vi "escalon_lab2.vi"() -> ()   [LabVIEW 2025]
uses:
  <vilib>/Utility/file.llb/Write Delimited Spreadsheet (DBL).vi
panel:
  out "Numeric 2":dbl
  out "Numeric":dbl
  in  "DC":dbl
  out "Waveform Chart":dynamicdata(graph)
  out "Thermometer":dbl(slide) scale=0.0..100.0
  in  "stop":bool
  # "Duty Cycle [%]"
  # "ALTO:"
  # "BAJO:"
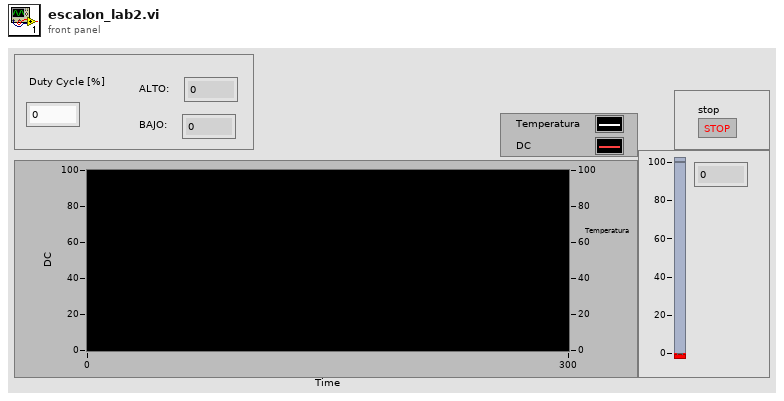
[diagram p1: front panel]
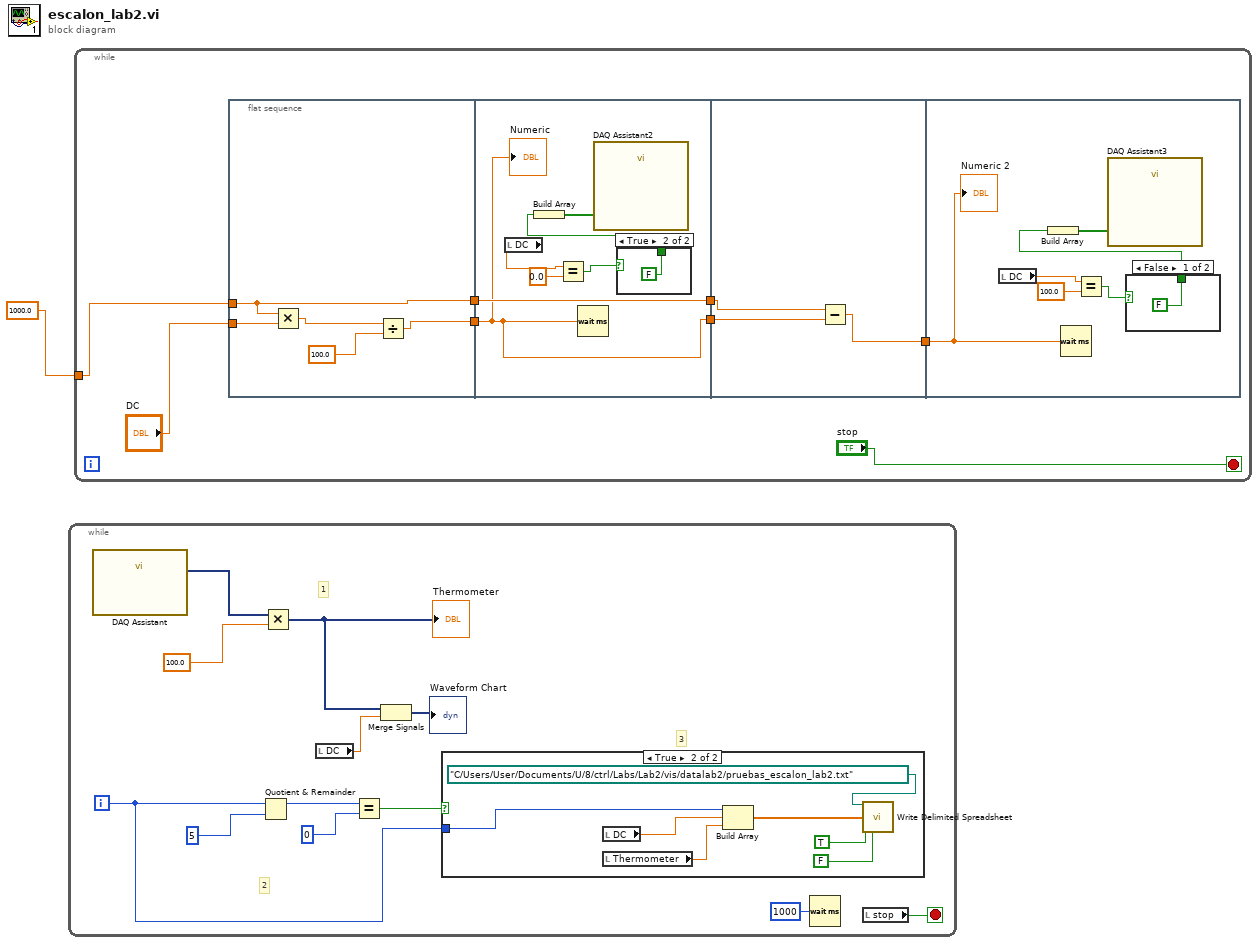
[diagram p0: block diagram]
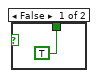
[diagram p2: hidden frame]
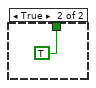
[diagram p3: hidden frame]
diagram:
  n1 = while {
    i -> [w6]
    stop <- w11 stop-if-true
    # "3"
    # "2"
    # "1"
    n2 = call "DAQ Assistant"() -> ("data"=w13:dynamicdata)  [unwired: 17 in, 2 out]
    n3 = Quotient & Remainder(x=w6, y=5) -> (x-y*floor(x/y)=w8:i32)  [unwired: 1 out]
    n4 = Multiply(x=w13, y=100.0) -> (x*y=w3:dynamicdata)
    "Thermometer" <- w3
    n5 = local read "DC"() -> (w2:dbl)
    n6 = Equal?(x=w8, y=0) -> (x = y?=w5:bool)
    n7 = Merge Signals(w3, w2) -> (→"Waveform Chart":dynamicdata)
    n8 = case shown="True" w5 {
      tunnel: w6 -> [_ w15]
      frame False {
      }
      frame True {
        n9 = local read "DC"() -> (w17:dbl)
        n10 = local read "Thermometer"() -> (w16:dbl)
        n11 = Build Array(w15, w17, w16) -> (w14:dbl[])
        n12 = call-poly <vilib>:"Write Delimited Spreadsheet.vi"("file path (dialog if empty)"=path "C:/Users/User/Documents/U/8/ctrl/Labs/Lab2/vis/datalab2/pruebas_escalon_lab2.txt", "1D data"=w14, "append to file? (new file:F)"=TRUE, "transpose? (no:F)"=FALSE) -> ()  [unwired: 10 in, 2 out]
      }
    }
    n13 = Wait (ms)(milliseconds to wait=u32 1000) -> ()  [unwired: 1 out]
    n14 = local read "stop"() -> (w11:bool)
  }
  n15 = while {
    tunnel: 1000.0 -> [w27]
    stop <- "stop" stop-if-true
    n16 = flat-sequence {
      tunnel: "DC" -> [w33]
      tunnel: w27 -> [w29]
      tunnel: [w30] -> w26
      tunnel: [w29] -> w25
      tunnel: w26 -> [w38]
      tunnel: w25 -> [w39]
      tunnel: [w39] -> w24
      tunnel: [w38] -> w23
      tunnel: w24 -> [w45]
      tunnel: w23 -> [w44]
      tunnel: [w43] -> w22
      tunnel: w22 -> [w50]
      frame #0 {
        n17 = Multiply(x=w29, y=w33) -> (x*y=w32:dbl)
        n18 = Divide(x=w32, y=100.0) -> (x/y=w30:dbl)
      }
      frame #1 {
        n19 = local read "DC"() -> (w37:dbl)
        n20 = Equal?(x=w37, y=0.0) -> (x = y?=w35:bool)
        n21 = Wait (ms)(milliseconds to wait=w38) -> ()  [unwired: 1 out]
        n22 = case shown="True" w35 {
          tunnel: [TRUE FALSE] -> w34
          frame False {
          }
          frame True {
          }
        }
        n23 = Build Array(w34) -> (w40:bool[])
        n24 = call "DAQ Assistant2"("data"=w40) -> ()  [unwired: 17 in, 2 out]
        "Numeric" <- w38
      }
      frame #2 {
        n25 = Subtract(x=w45, y=w44) -> (x-y=w43:dbl)
      }
      frame #3 {
        n26 = local read "DC"() -> (w49:dbl)
        n27 = Wait (ms)(milliseconds to wait=w50) -> ()  [unwired: 1 out]
        n28 = Equal?(x=w49, y=100.0) -> (x = y?=w47:bool)
        n29 = case shown="False" w47 {
          tunnel: [FALSE TRUE] -> w46
          frame False {
          }
          frame True {
          }
        }
        n30 = Build Array(w46) -> (w51:bool[])
        n31 = call "DAQ Assistant3"("data"=w51) -> ()  [unwired: 17 in, 2 out]
        "Numeric 2" <- w50
      }
    }
  }
